vi "RegPatchGenerator.vi"(8 "error in":errorcluster, 9 "reg patch file":path=path "C:/Users/liyao/Desktop", 10 "extensions":string[](array[string])=[".lvproj", ".lvlib", ".lvlibp", ".vi", ".llb", ".ctl", ".lvclass", ".vit", ".xctl", ".lvsc", ".lvrbt", ".vim", ".lvtest", ".ctt"], 11 "exe path":path=path "C:/Users/liyao/Desktop/LabVIEW-Version-Selector/Build/LabVIEW Version Selector.exe") -> (0 "error out":errorcluster, 3 "install.reg":string="Windows Registry Editor Version 5.00\n\n[HKEY_CLASSES_ROOT\\Applications\\LabVIEW Version Selector.exe]\n\n[HKEY_CLASSES_ROOT\\Applications\\LabVIEW Version Selector.exe\\shell]\n\n[HKEY_CLASSES_ROOT\\Applications\\LabVIEW Version Selector.exe\\shell\\open]\n\n[HKEY_CLASSES_ROOT\\Applications\\LabVIEW Version Selector.exe\\shell\\open\\command]\n@=\"\\\"\"\"\" \"%1\"\"\\\" \\\"%1\\\"\"\n\n[HKEY_CURRENT_USER\\Software\\Classes\\Applications\\LabVIEW Version Selector.exe]\n\n[HKEY_CURRENT_USER\\Software\\Classes\\Applications\\LabVIEW Version Selector.exe\\shell]\n\n[HKEY_CURRENT_USER\\Software\\Classes\\Applications\\LabVIEW Version Selector.exe\\shell\\open]\n\n[HKEY_CURRENT_USER\\Software\\Classes\\Applications\\LabVIEW Version Selector.exe\\shell\\open\\command]\n@=\"\\\"\"\"\" \"%1\"\"\\\" \\\"%1\\\"\"\n\n[HKEY_CURRENT_USER\\Software\\Microsoft\\Windows\\CurrentVersion\\Explorer\\FileExts\\.lvproj\\OpenWithList]\n\"a\"=\"LabVIEW.exe\"\n\"b\"=\"LabVIEW Version Selector.exe\"\n\"MRUList\"=\"ba\"\n\n[HKEY_CURRENT_USER\\Software\\Microsoft\\Windows\\CurrentVersion\\Explorer\\FileExts\\.lvproj\\UserChoice]\n\"ProgId\"=\"Applications\\\\LabVIEW Version Selector.exe\"\n\n[HKEY_CLASSES_ROOT\\LabVIEWProject\r\n\\shell\\open\\command]\n@=\"\\\"\"\"\" \"%1\"\"\\\" \\\"%1\\\"\"\n\n[HKEY_LOCAL_MACHINE\\SOFTWARE\\Classes\\LabVIEWProject\r\n\\shell\\open\\command]\n@=hex(2):<HEXEXEPATH>\n\n[HKEY_CURRENT_USER\\Software\\Microsoft\\Windows\\CurrentVersion\\Explorer\\FileExts\\.lvlib\\OpenWithList]\n\"a\"=\"LabVIEW.exe\"\n\"b\"=\"LabVIEW Version Selector.exe\"\n\"MRUList\"=\"ba\"\n\n[HKEY_CURRENT_USER\\Software\\Microsoft\\Windows\\CurrentVersion\\Explorer\\FileExts\\.lvlib\\UserChoice]\n\"ProgId\"=\"Applications\\\\LabVIEW Version Selector.exe\"\n\n[HKEY_CLASSES_ROOT\\LabVIEWLabVIEW Library\r\n\\shell\\open\\command]\n@=\"\\\"\"\"\" \"%1\"\"\\\" \\\"%1\\\"\"\n\n[HKEY_LOCAL_MACHINE\\SOFTWARE\\Classes\\LabVIEWLabVIEW Library\r\n\\shell\\open\\command]\n@=hex(2):<HEXEXEPATH>\n\n[HKEY_CURRENT_USER\\Software\\Microsoft\\Windows\\CurrentVersion\\Explorer\\FileExts\\.lvlibp\\OpenWithList]\n\"a\"=\"LabVIEW.exe\"\n\"b\"=\"LabVIEW Version Selector.exe\"\n\"MRUList\"=\"ba\"\n\n[HKEY_CURRENT_USER\\Software\\Microsoft\\Windows\\CurrentVersion\\Explorer\\FileExts\\.lvlibp\\UserChoice]\n\"ProgId\"=\"Applications\\\\LabVIEW Version Selector.exe\"\n\n[HKEY_CLASSES_ROOT\\LabVIEWLabVIEW Packed Library\r\n\\shell\\open\\command]\n@=\"\\\"\"\"\" \"%1\"\"\\\" \\\"%1\\\"\"\n\n[HKEY_LOCAL_MACHINE\\SOFTWARE\\Classes\\LabVIEWLabVIEW Packed Library\r\n\\shell\\open\\command]\n@=hex(2):<HEXEXEPATH>\n\n[HKEY_CURRENT_USER\\Software\\Microsoft\\Windows\\CurrentVersion\\Explorer\\FileExts\\.vi\\OpenWithList]\n\"a\"=\"LabVIEW.exe\"\n\"b\"=\"LabVIEW Version Selector.exe\"\n\"MRUList\"=\"ba\"\n\n[HKEY_CURRENT_USER\\Software\\Microsoft\\Windows\\CurrentVersion\\Explorer\\FileExts\\.vi\\UserChoice]\n\"ProgId\"=\"Applications\\\\LabVIEW Version Selector.exe\"\n\n[HKEY_CLASSES_ROOT\\LabVIEWInstrument\r\n\\shell\\open\\command]\n@=\"\\\"\"\"\" \"%1\"\"\\\" \\\"%1\\\"\"\n\n[HKEY_LOCAL_MACHINE\\SOFTWARE\\Classes\\LabVIEWInstrument\r\n\\shell\\open\\command]\n@=hex(2):<HEXEXEPATH>\n\n[HKEY_CURRENT_USER\\Software\\Microsoft\\Windows\\CurrentVersion\\Explorer\\FileExts\\.llb\\OpenWithList]\n\"a\"=\"LabVIEW.exe\"\n\"b\"=\"LabVIEW Version Selector.exe\"\n\"MRUList\"=\"ba\"\n\n[HKEY_CURRENT_USER\\Software\\Microsoft\\Windows\\CurrentVersion\\Explorer\\FileExts\\.llb\\UserChoice]\n\"ProgId\"=\"Applications\\\\LabVIEW Version Selector.exe\"\n\n[HKEY_CLASSES_ROOT\\LabVIEWLibrary\r\n\\shell\\open\\command]\n@=\"\\\"\"\"\" \"%1\"\"\\\" \\\"%1\\\"\"\n\n[HKEY_LOCAL_MACHINE\\SOFTWARE\\Classes\\LabVIEWLibrary\r\n\\shell\\open\\command]\n@=hex(2):<HEXEXEPATH>\n\n[HKEY_CURRENT_USER\\Software\\Microsoft\\Windows\\CurrentVersion\\Explorer\\FileExts\\.ctl\\OpenWithList]\n\"a\"=\"LabVIEW.exe\"\n\"b\"=\"LabVIEW Version Selector.exe\"\n\"MRUList\"=\"ba\"\n\n[HKEY_CURRENT_USER\\Software\\Microsoft\\Windows\\CurrentVersion\\Explorer\\FileExts\\.ctl\\UserChoice]\n\"ProgId\"=\"Applications\\\\LabVIEW Version Selector.exe\"\n\n[HKEY_CLASSES_ROOT\\LabVIEWControl\r\n\\shell\\open\\command]\n@=\"\\\"\"\"\" \"%1\"\"\\\" \\\"%1\\\"\"\n\n[HKEY_LOCAL_MACHINE\\SOFTWARE\\Classes\\LabVIEWControl\r\n\\shell\\open\\command]\n@=hex(2):<HEXEXEPATH>\n\n[HKEY_CURRENT_USER\\Software\\Microsoft\\Windows\\CurrentVersion\\Explorer\\FileExts\\.lvclass\\OpenWithList]\n\"a\"=\"LabVIEW.exe\"\n\"b\"=\"LabVIEW Version Selector.exe\"\n\"MRUList\"=\"ba\"\n\n[HKEY_CURRENT_USER\\Software\\Microsoft\\Windows\\CurrentVersion\\Explorer\\FileExts\\.lvclass\\UserChoice]\n\"ProgId\"=\"Applications\\\\LabVIEW Version Selector.exe\"\n\n[HKEY_CLASSES_ROOT\\LabVIEWLabVIEW Class\r\n\\shell\\open\\command]\n@=\"\\\"\"\"\" \"%1\"\"\\\" \\\"%1\\\"\"\n\n[HKEY_LOCAL_MACHINE\\SOFTWARE\\Classes\\LabVIEWLabVIEW Class\r\n\\shell\\open\\command]\n@=hex(2):<HEXEXEPATH>\n\n[HKEY_CURRENT_USER\\Software\\Microsoft\\Windows\\CurrentVersion\\Explorer\\FileExts\\.vit\\OpenWithList]\n\"a\"=\"LabVIEW.exe\"\n\"b\"=\"LabVIEW Version Selector.exe\"\n\"MRUList\"=\"ba\"\n\n[HKEY_CURRENT_USER\\Software\\Microsoft\\Windows\\CurrentVersion\\Explorer\\FileExts\\.vit\\UserChoice]\n\"ProgId\"=\"Applications\\\\LabVIEW Version Selector.exe\"\n\n[HKEY_CLASSES_ROOT\\LabVIEWInstrumentTemplate\r\n\\shell\\open\\command]\n@=\"\\\"\"\"\" \"%1\"\"\\\" \\\"%1\\\"\"\n\n[HKEY_LOCAL_MACHINE\\SOFTWARE\\Classes\\LabVIEWInstrumentTemplate\r\n\\shell\\open\\command]\n@=hex(2):<HEXEXEPATH>\n\n[HKEY_CURRENT_USER\\Software\\Microsoft\\Windows\\CurrentVersion\\Explorer\\FileExts\\.xctl\\OpenWithList]\n\"a\"=\"LabVIEW.exe\"\n\"b\"=\"LabVIEW Version Selector.exe\"\n\"MRUList\"=\"ba\"\n\n[HKEY_CURRENT_USER\\Software\\Microsoft\\Windows\\CurrentVersion\\Explorer\\FileExts\\.xctl\\UserChoice]\n\"ProgId\"=\"Applications\\\\LabVIEW Version Selector.exe\"\n\n[HKEY_CLASSES_ROOT\\LabVIEWXControl\r\n\\shell\\open\\command]\n@=\"\\\"\"\"\" \"%1\"\"\\\" \\\"%1\\\"\"\n\n[HKEY_LOCAL_MACHINE\\SOFTWARE\\Classes\\LabVIEWXControl\r\n\\shell\\open\\command]\n@=hex(2):<HEXEXEPATH>\n\n[HKEY_CURRENT_USER\\Software\\Microsoft\\Windows\\CurrentVersion\\Explorer\\FileExts\\.lvtest\\OpenWithList]\n\"a\"=\"LabVIEW.exe\"\n\"b\"=\"LabVIEW Version Selector.exe\"\n\"MRUList\"=\"ba\"\n\n[HKEY_CURRENT_USER\\Software\\Microsoft\\Windows\\CurrentVersion\\Explorer\\FileExts\\.lvtest\\UserChoice]\n\"ProgId\"=\"Applications\\\\LabVIEW Version Selector.exe\"\n\n[HKEY_CLASSES_ROOT\\\\shell\\open\\command]\n@=\"\\\"\"\"\" \"%1\"\"\\\" \\\"%1\\\"\"\n\n[HKEY_LOCAL_MACHINE\\SOFTWARE\\Classes\\\\shell\\open\\command]\n@=hex(2):<HEXEXEPATH>\n\n[HKEY_CURRENT_USER\\Software\\Microsoft\\Windows\\CurrentVersion\\Explorer\\FileExts\\.lvvect\\OpenWithList]\n\"a\"=\"LabVIEW.exe\"\n\"b\"=\"LabVIEW Version Selector.exe\"\n\"MRUList\"=\"ba\"\n\n[HKEY_CURRENT_USER\\Software\\Microsoft\\Windows\\CurrentVersion\\Explorer\\FileExts\\.lvvect\\UserChoice]\n\"ProgId\"=\"Applications\\\\LabVIEW Version Selector.exe\"\n\n[HKEY_CLASSES_ROOT\\\\shell\\open\\command]\n@=\"\\\"\"\"\" \"%1\"\"\\\" \\\"%1\\\"\"\n\n[HKEY_LOCAL_MACHINE\\SOFTWARE\\Classes\\\\shell\\open\\command]\n@=hex(2):<HEXEXEPATH>\n\n[HKEY_CURRENT_USER\\Software\\Microsoft\\Windows\\CurrentVersion\\Explorer\\FileExts\\.lvsc\\OpenWithList]\n\"a\"=\"LabVIEW.exe\"\n\"b\"=\"LabVIEW Version Selector.exe\"\n\"MRUList\"=\"ba\"\n\n[HKEY_CURRENT_USER\\Software\\Microsoft\\Windows\\CurrentVersion\\Explorer\\FileExts\\.lvsc\\UserChoice]\n\"ProgId\"=\"Applications\\\\LabVIEW Version Selector.exe\"\n\n[HKEY_CLASSES_ROOT\\LabVIEW Statechart\r\n\\shell\\open\\command]\n@=\"\\\"\"\"\" \"%1\"\"\\\" \\\"%1\\\"\"\n\n[HKEY_LOCAL_MACHINE\\SOFTWARE\\Classes\\LabVIEW Statechart\r\n\\shell\\open\\command]\n@=hex(2):<HEXEXEPATH>\n\n[HKEY_CURRENT_USER\\Software\\Microsoft\\Windows\\CurrentVersion\\Explorer\\FileExts\\.LVCLASS\\OpenWithList]\n\"a\"=\"LabVIEW.exe\"\n\"b\"=\"LabVIEW Version Selector.exe\"\n\"MRUList\"=\"ba\"\n\n[HKEY_CURRENT_USER\\Software\\Microsoft\\Windows\\CurrentVersion\\Explorer\\FileExts\\.LVCLASS\\UserChoice]\n\"ProgId\"=\"Applications\\\\LabVIEW Version Selector.exe\"\n\n[HKEY_CLASSES_ROOT\\LabVIEWLabVIEW Class\r\n\\shell\\open\\command]\n@=\"\\\"\"\"\" \"%1\"\"\\\" \\\"%1\\\"\"\n\n[HKEY_LOCAL_MACHINE\\SOFTWARE\\Classes\\LabVIEWLabVIEW Class\r\n\\shell\\open\\command]\n@=hex(2):<HEXEXEPATH>\n\n[HKEY_CURRENT_USER\\Software\\Microsoft\\Windows\\CurrentVersion\\Explorer\\FileExts\\.lvr\\OpenWithList]\n\"a\"=\"LabVIEW.exe\"\n\"b\"=\"LabVIEW Version Selector.exe\"\n\"MRUList\"=\"ba\"\n\n[HKEY_CURRENT_USER\\Software\\Microsoft\\Windows\\CurrentVersion\\Explorer\\FileExts\\.lvr\\UserChoice]\n\"ProgId\"=\"Applications\\\\LabVIEW Version Selector.exe\"\n\n[HKEY_CLASSES_ROOT\\\\shell\\open\\command]\n@=\"\\\"\"\"\" \"%1\"\"\\\" \\\"%1\\\"\"\n\n[HKEY_LOCAL_MACHINE\\SOFTWARE\\Classes\\\\shell\\open\\command]\n@=hex(2):<HEXEXEPATH>\n\n[HKEY_CURRENT_USER\\Software\\Microsoft\\Windows\\CurrentVersion\\Explorer\\FileExts\\.lvrbt\\OpenWithList]\n\"a\"=\"LabVIEW.exe\"\n\"b\"=\"LabVIEW Version Selector.exe\"\n\"MRUList\"=\"ba\"\n\n[HKEY_CURRENT_USER\\Software\\Microsoft\\Windows\\CurrentVersion\\Explorer\\FileExts\\.lvrbt\\UserChoice]\n\"ProgId\"=\"Applications\\\\LabVIEW Version Selector.exe\"\n\n[HKEY_CLASSES_ROOT\\LabVIEWNXTRobotProject\r\n\\shell\\open\\command]\n@=\"\\\"\"\"\" \"%1\"\"\\\" \\\"%1\\\"\"\n\n[HKEY_LOCAL_MACHINE\\SOFTWARE\\Classes\\LabVIEWNXTRobotProject\r\n\\shell\\open\\command]\n@=hex(2):<HEXEXEPATH>")   [LabVIEW 2014]
uses:
  <userlib>/_OpenG.lib/array/array.llb/Remove Duplicates from 1D Array (String)__ogtk.vi
panel:
  out "unstall.reg":string="Windows Registry Editor Version 5.00\n\n[HKEY_CLASSES_ROOT\\Applications\\LabVIEW Version Selector.exe]\n\n[HKEY_CLASSES_ROOT\\Applications\\LabVIEW Version Selector.exe\\shell]\n\n[HKEY_CLASSES_ROOT\\Applications\\LabVIEW Version Selector.exe\\shell\\open]\n\n[HKEY_CLASSES_ROOT\\Applications\\LabVIEW Version Selector.exe\\shell\\open\\command]\n@=\"\\\"\"\"\" \"%1\"\"\\\" \\\"%1\\\"\"\n\n[HKEY_CURRENT_USER\\Software\\Classes\\Applications\\LabVIEW Version Selector.exe]\n\n[HKEY_CURRENT_USER\\Software\\Classes\\Applications\\LabVIEW Version Selector.exe\\shell]\n\n[HKEY_CURRENT_USER\\Software\\Classes\\Applications\\LabVIEW Version Selector.exe\\shell\\open]\n\n[HKEY_CURRENT_USER\\Software\\Classes\\Applications\\LabVIEW Version Selector.exe\\shell\\open\\command]\n@=\"\\\"\"\"\" \"%1\"\"\\\" \\\"%1\\\"\"\n\n[HKEY_CURRENT_USER\\Software\\Microsoft\\Windows\\CurrentVersion\\Explorer\\FileExts\\.lvproj\\OpenWithList]\n\"a\"=\"LabVIEW.exe\"\n\"b\"=\"LabVIEW Version Selector.exe\"\n\"MRUList\"=\"ba\"\n\n[HKEY_CURRENT_USER\\Software\\Microsoft\\Windows\\CurrentVersion\\Explorer\\FileExts\\.lvproj\\UserChoice]\n\"ProgId\"=\"Applications\\\\LabVIEW Version Selector.exe\"\n\n[HKEY_CLASSES_ROOT\\LabVIEWProject\r\n\\shell\\open\\command]\n@=\"\\\"\"\"\" \"%1\"\"\\\" \\\"%1\\\"\"\n\n[HKEY_LOCAL_MACHINE\\SOFTWARE\\Classes\\LabVIEWProject\r\n\\shell\\open\\command]\n@=hex(2):<HEXEXEPATH>\n\n[HKEY_CURRENT_USER\\Software\\Microsoft\\Windows\\CurrentVersion\\Explorer\\FileExts\\.lvlib\\OpenWithList]\n\"a\"=\"LabVIEW.exe\"\n\"b\"=\"LabVIEW Version Selector.exe\"\n\"MRUList\"=\"ba\"\n\n[HKEY_CURRENT_USER\\Software\\Microsoft\\Windows\\CurrentVersion\\Explorer\\FileExts\\.lvlib\\UserChoice]\n\"ProgId\"=\"Applications\\\\LabVIEW Version Selector.exe\"\n\n[HKEY_CLASSES_ROOT\\LabVIEWLabVIEW Library\r\n\\shell\\open\\command]\n@=\"\\\"\"\"\" \"%1\"\"\\\" \\\"%1\\\"\"\n\n[HKEY_LOCAL_MACHINE\\SOFTWARE\\Classes\\LabVIEWLabVIEW Library\r\n\\shell\\open\\command]\n@=hex(2):<HEXEXEPATH>\n\n[HKEY_CURRENT_USER\\Software\\Microsoft\\Windows\\CurrentVersion\\Explorer\\FileExts\\.lvlibp\\OpenWithList]\n\"a\"=\"LabVIEW.exe\"\n\"b\"=\"LabVIEW Version Selector.exe\"\n\"MRUList\"=\"ba\"\n\n[HKEY_CURRENT_USER\\Software\\Microsoft\\Windows\\CurrentVersion\\Explorer\\FileExts\\.lvlibp\\UserChoice]\n\"ProgId\"=\"Applications\\\\LabVIEW Version Selector.exe\"\n\n[HKEY_CLASSES_ROOT\\LabVIEWLabVIEW Packed Library\r\n\\shell\\open\\command]\n@=\"\\\"\"\"\" \"%1\"\"\\\" \\\"%1\\\"\"\n\n[HKEY_LOCAL_MACHINE\\SOFTWARE\\Classes\\LabVIEWLabVIEW Packed Library\r\n\\shell\\open\\command]\n@=hex(2):<HEXEXEPATH>\n\n[HKEY_CURRENT_USER\\Software\\Microsoft\\Windows\\CurrentVersion\\Explorer\\FileExts\\.vi\\OpenWithList]\n\"a\"=\"LabVIEW.exe\"\n\"b\"=\"LabVIEW Version Selector.exe\"\n\"MRUList\"=\"ba\"\n\n[HKEY_CURRENT_USER\\Software\\Microsoft\\Windows\\CurrentVersion\\Explorer\\FileExts\\.vi\\UserChoice]\n\"ProgId\"=\"Applications\\\\LabVIEW Version Selector.exe\"\n\n[HKEY_CLASSES_ROOT\\LabVIEWInstrument\r\n\\shell\\open\\command]\n@=\"\\\"\"\"\" \"%1\"\"\\\" \\\"%1\\\"\"\n\n[HKEY_LOCAL_MACHINE\\SOFTWARE\\Classes\\LabVIEWInstrument\r\n\\shell\\open\\command]\n@=hex(2):<HEXEXEPATH>\n\n[HKEY_CURRENT_USER\\Software\\Microsoft\\Windows\\CurrentVersion\\Explorer\\FileExts\\.llb\\OpenWithList]\n\"a\"=\"LabVIEW.exe\"\n\"b\"=\"LabVIEW Version Selector.exe\"\n\"MRUList\"=\"ba\"\n\n[HKEY_CURRENT_USER\\Software\\Microsoft\\Windows\\CurrentVersion\\Explorer\\FileExts\\.llb\\UserChoice]\n\"ProgId\"=\"Applications\\\\LabVIEW Version Selector.exe\"\n\n[HKEY_CLASSES_ROOT\\LabVIEWLibrary\r\n\\shell\\open\\command]\n@=\"\\\"\"\"\" \"%1\"\"\\\" \\\"%1\\\"\"\n\n[HKEY_LOCAL_MACHINE\\SOFTWARE\\Classes\\LabVIEWLibrary\r\n\\shell\\open\\command]\n@=hex(2):<HEXEXEPATH>\n\n[HKEY_CURRENT_USER\\Software\\Microsoft\\Windows\\CurrentVersion\\Explorer\\FileExts\\.ctl\\OpenWithList]\n\"a\"=\"LabVIEW.exe\"\n\"b\"=\"LabVIEW Version Selector.exe\"\n\"MRUList\"=\"ba\"\n\n[HKEY_CURRENT_USER\\Software\\Microsoft\\Windows\\CurrentVersion\\Explorer\\FileExts\\.ctl\\UserChoice]\n\"ProgId\"=\"Applications\\\\LabVIEW Version Selector.exe\"\n\n[HKEY_CLASSES_ROOT\\LabVIEWControl\r\n\\shell\\open\\command]\n@=\"\\\"\"\"\" \"%1\"\"\\\" \\\"%1\\\"\"\n\n[HKEY_LOCAL_MACHINE\\SOFTWARE\\Classes\\LabVIEWControl\r\n\\shell\\open\\command]\n@=hex(2):<HEXEXEPATH>\n\n[HKEY_CURRENT_USER\\Software\\Microsoft\\Windows\\CurrentVersion\\Explorer\\FileExts\\.lvclass\\OpenWithList]\n\"a\"=\"LabVIEW.exe\"\n\"b\"=\"LabVIEW Version Selector.exe\"\n\"MRUList\"=\"ba\"\n\n[HKEY_CURRENT_USER\\Software\\Microsoft\\Windows\\CurrentVersion\\Explorer\\FileExts\\.lvclass\\UserChoice]\n\"ProgId\"=\"Applications\\\\LabVIEW Version Selector.exe\"\n\n[HKEY_CLASSES_ROOT\\LabVIEWLabVIEW Class\r\n\\shell\\open\\command]\n@=\"\\\"\"\"\" \"%1\"\"\\\" \\\"%1\\\"\"\n\n[HKEY_LOCAL_MACHINE\\SOFTWARE\\Classes\\LabVIEWLabVIEW Class\r\n\\shell\\open\\command]\n@=hex(2):<HEXEXEPATH>\n\n[HKEY_CURRENT_USER\\Software\\Microsoft\\Windows\\CurrentVersion\\Explorer\\FileExts\\.vit\\OpenWithList]\n\"a\"=\"LabVIEW.exe\"\n\"b\"=\"LabVIEW Version Selector.exe\"\n\"MRUList\"=\"ba\"\n\n[HKEY_CURRENT_USER\\Software\\Microsoft\\Windows\\CurrentVersion\\Explorer\\FileExts\\.vit\\UserChoice]\n\"ProgId\"=\"Applications\\\\LabVIEW Version Selector.exe\"\n\n[HKEY_CLASSES_ROOT\\LabVIEWInstrumentTemplate\r\n\\shell\\open\\command]\n@=\"\\\"\"\"\" \"%1\"\"\\\" \\\"%1\\\"\"\n\n[HKEY_LOCAL_MACHINE\\SOFTWARE\\Classes\\LabVIEWInstrumentTemplate\r\n\\shell\\open\\command]\n@=hex(2):<HEXEXEPATH>\n\n[HKEY_CURRENT_USER\\Software\\Microsoft\\Windows\\CurrentVersion\\Explorer\\FileExts\\.xctl\\OpenWithList]\n\"a\"=\"LabVIEW.exe\"\n\"b\"=\"LabVIEW Version Selector.exe\"\n\"MRUList\"=\"ba\"\n\n[HKEY_CURRENT_USER\\Software\\Microsoft\\Windows\\CurrentVersion\\Explorer\\FileExts\\.xctl\\UserChoice]\n\"ProgId\"=\"Applications\\\\LabVIEW Version Selector.exe\"\n\n[HKEY_CLASSES_ROOT\\LabVIEWXControl\r\n\\shell\\open\\command]\n@=\"\\\"\"\"\" \"%1\"\"\\\" \\\"%1\\\"\"\n\n[HKEY_LOCAL_MACHINE\\SOFTWARE\\Classes\\LabVIEWXControl\r\n\\shell\\open\\command]\n@=hex(2):<HEXEXEPATH>\n\n[HKEY_CURRENT_USER\\Software\\Microsoft\\Windows\\CurrentVersion\\Explorer\\FileExts\\.lvtest\\OpenWithList]\n\"a\"=\"LabVIEW.exe\"\n\"b\"=\"LabVIEW Version Selector.exe\"\n\"MRUList\"=\"ba\"\n\n[HKEY_CURRENT_USER\\Software\\Microsoft\\Windows\\CurrentVersion\\Explorer\\FileExts\\.lvtest\\UserChoice]\n\"ProgId\"=\"Applications\\\\LabVIEW Version Selector.exe\"\n\n[HKEY_CLASSES_ROOT\\\\shell\\open\\command]\n@=\"\\\"\"\"\" \"%1\"\"\\\" \\\"%1\\\"\"\n\n[HKEY_LOCAL_MACHINE\\SOFTWARE\\Classes\\\\shell\\open\\command]\n@=hex(2):<HEXEXEPATH>\n\n[HKEY_CURRENT_USER\\Software\\Microsoft\\Windows\\CurrentVersion\\Explorer\\FileExts\\.lvvect\\OpenWithList]\n\"a\"=\"LabVIEW.exe\"\n\"b\"=\"LabVIEW Version Selector.exe\"\n\"MRUList\"=\"ba\"\n\n[HKEY_CURRENT_USER\\Software\\Microsoft\\Windows\\CurrentVersion\\Explorer\\FileExts\\.lvvect\\UserChoice]\n\"ProgId\"=\"Applications\\\\LabVIEW Version Selector.exe\"\n\n[HKEY_CLASSES_ROOT\\\\shell\\open\\command]\n@=\"\\\"\"\"\" \"%1\"\"\\\" \\\"%1\\\"\"\n\n[HKEY_LOCAL_MACHINE\\SOFTWARE\\Classes\\\\shell\\open\\command]\n@=hex(2):<HEXEXEPATH>\n\n[HKEY_CURRENT_USER\\Software\\Microsoft\\Windows\\CurrentVersion\\Explorer\\FileExts\\.lvsc\\OpenWithList]\n\"a\"=\"LabVIEW.exe\"\n\"b\"=\"LabVIEW Version Selector.exe\"\n\"MRUList\"=\"ba\"\n\n[HKEY_CURRENT_USER\\Software\\Microsoft\\Windows\\CurrentVersion\\Explorer\\FileExts\\.lvsc\\UserChoice]\n\"ProgId\"=\"Applications\\\\LabVIEW Version Selector.exe\"\n\n[HKEY_CLASSES_ROOT\\LabVIEW Statechart\r\n\\shell\\open\\command]\n@=\"\\\"\"\"\" \"%1\"\"\\\" \\\"%1\\\"\"\n\n[HKEY_LOCAL_MACHINE\\SOFTWARE\\Classes\\LabVIEW Statechart\r\n\\shell\\open\\command]\n@=hex(2):<HEXEXEPATH>\n\n[HKEY_CURRENT_USER\\Software\\Microsoft\\Windows\\CurrentVersion\\Explorer\\FileExts\\.LVCLASS\\OpenWithList]\n\"a\"=\"LabVIEW.exe\"\n\"b\"=\"LabVIEW Version Selector.exe\"\n\"MRUList\"=\"ba\"\n\n[HKEY_CURRENT_USER\\Software\\Microsoft\\Windows\\CurrentVersion\\Explorer\\FileExts\\.LVCLASS\\UserChoice]\n\"ProgId\"=\"Applications\\\\LabVIEW Version Selector.exe\"\n\n[HKEY_CLASSES_ROOT\\LabVIEWLabVIEW Class\r\n\\shell\\open\\command]\n@=\"\\\"\"\"\" \"%1\"\"\\\" \\\"%1\\\"\"\n\n[HKEY_LOCAL_MACHINE\\SOFTWARE\\Classes\\LabVIEWLabVIEW Class\r\n\\shell\\open\\command]\n@=hex(2):<HEXEXEPATH>\n\n[HKEY_CURRENT_USER\\Software\\Microsoft\\Windows\\CurrentVersion\\Explorer\\FileExts\\.lvr\\OpenWithList]\n\"a\"=\"LabVIEW.exe\"\n\"b\"=\"LabVIEW Version Selector.exe\"\n\"MRUList\"=\"ba\"\n\n[HKEY_CURRENT_USER\\Software\\Microsoft\\Windows\\CurrentVersion\\Explorer\\FileExts\\.lvr\\UserChoice]\n\"ProgId\"=\"Applications\\\\LabVIEW Version Selector.exe\"\n\n[HKEY_CLASSES_ROOT\\\\shell\\open\\command]\n@=\"\\\"\"\"\" \"%1\"\"\\\" \\\"%1\\\"\"\n\n[HKEY_LOCAL_MACHINE\\SOFTWARE\\Classes\\\\shell\\open\\command]\n@=hex(2):<HEXEXEPATH>\n\n[HKEY_CURRENT_USER\\Software\\Microsoft\\Windows\\CurrentVersion\\Explorer\\FileExts\\.lvrbt\\OpenWithList]\n\"a\"=\"LabVIEW.exe\"\n\"b\"=\"LabVIEW Version Selector.exe\"\n\"MRUList\"=\"ba\"\n\n[HKEY_CURRENT_USER\\Software\\Microsoft\\Windows\\CurrentVersion\\Explorer\\FileExts\\.lvrbt\\UserChoice]\n\"ProgId\"=\"Applications\\\\LabVIEW Version Selector.exe\"\n\n[HKEY_CLASSES_ROOT\\LabVIEWNXTRobotProject\r\n\\shell\\open\\command]\n@=\"\\\"\"\"\" \"%1\"\"\\\" \\\"%1\\\"\"\n\n[HKEY_LOCAL_MACHINE\\SOFTWARE\\Classes\\LabVIEWNXTRobotProject\r\n\\shell\\open\\command]\n@=hex(2):<HEXEXEPATH>"
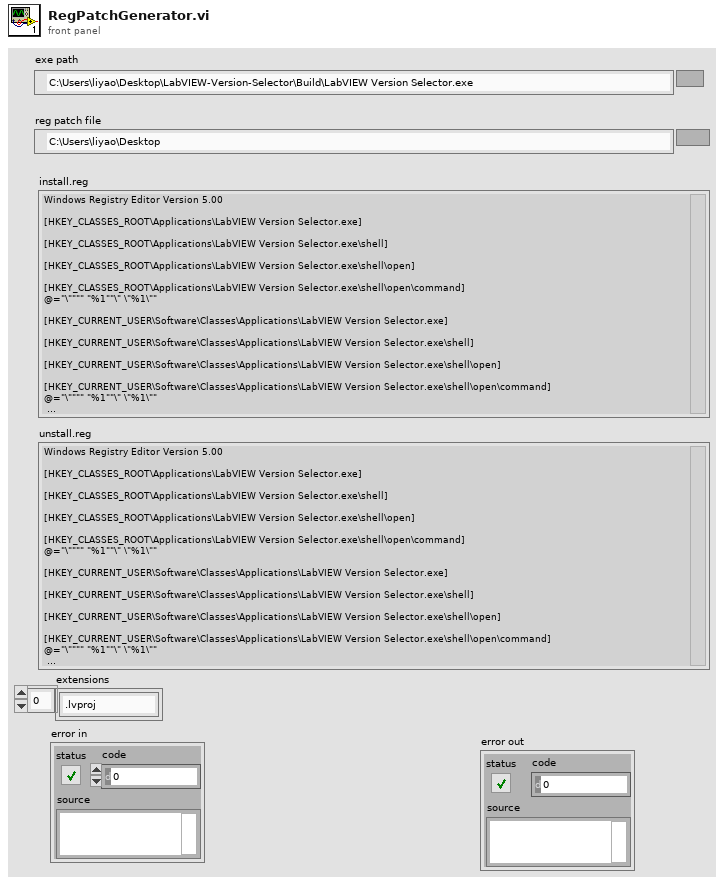
[diagram p1: front panel]
types:
  T1 = cluster{"dotEXT":string, "EXTTYPE":string[], "accoc":string}
  T2 = enum16{"open", "replace", "create", "open or create", "replace or create", "replace or create with confirmation"}
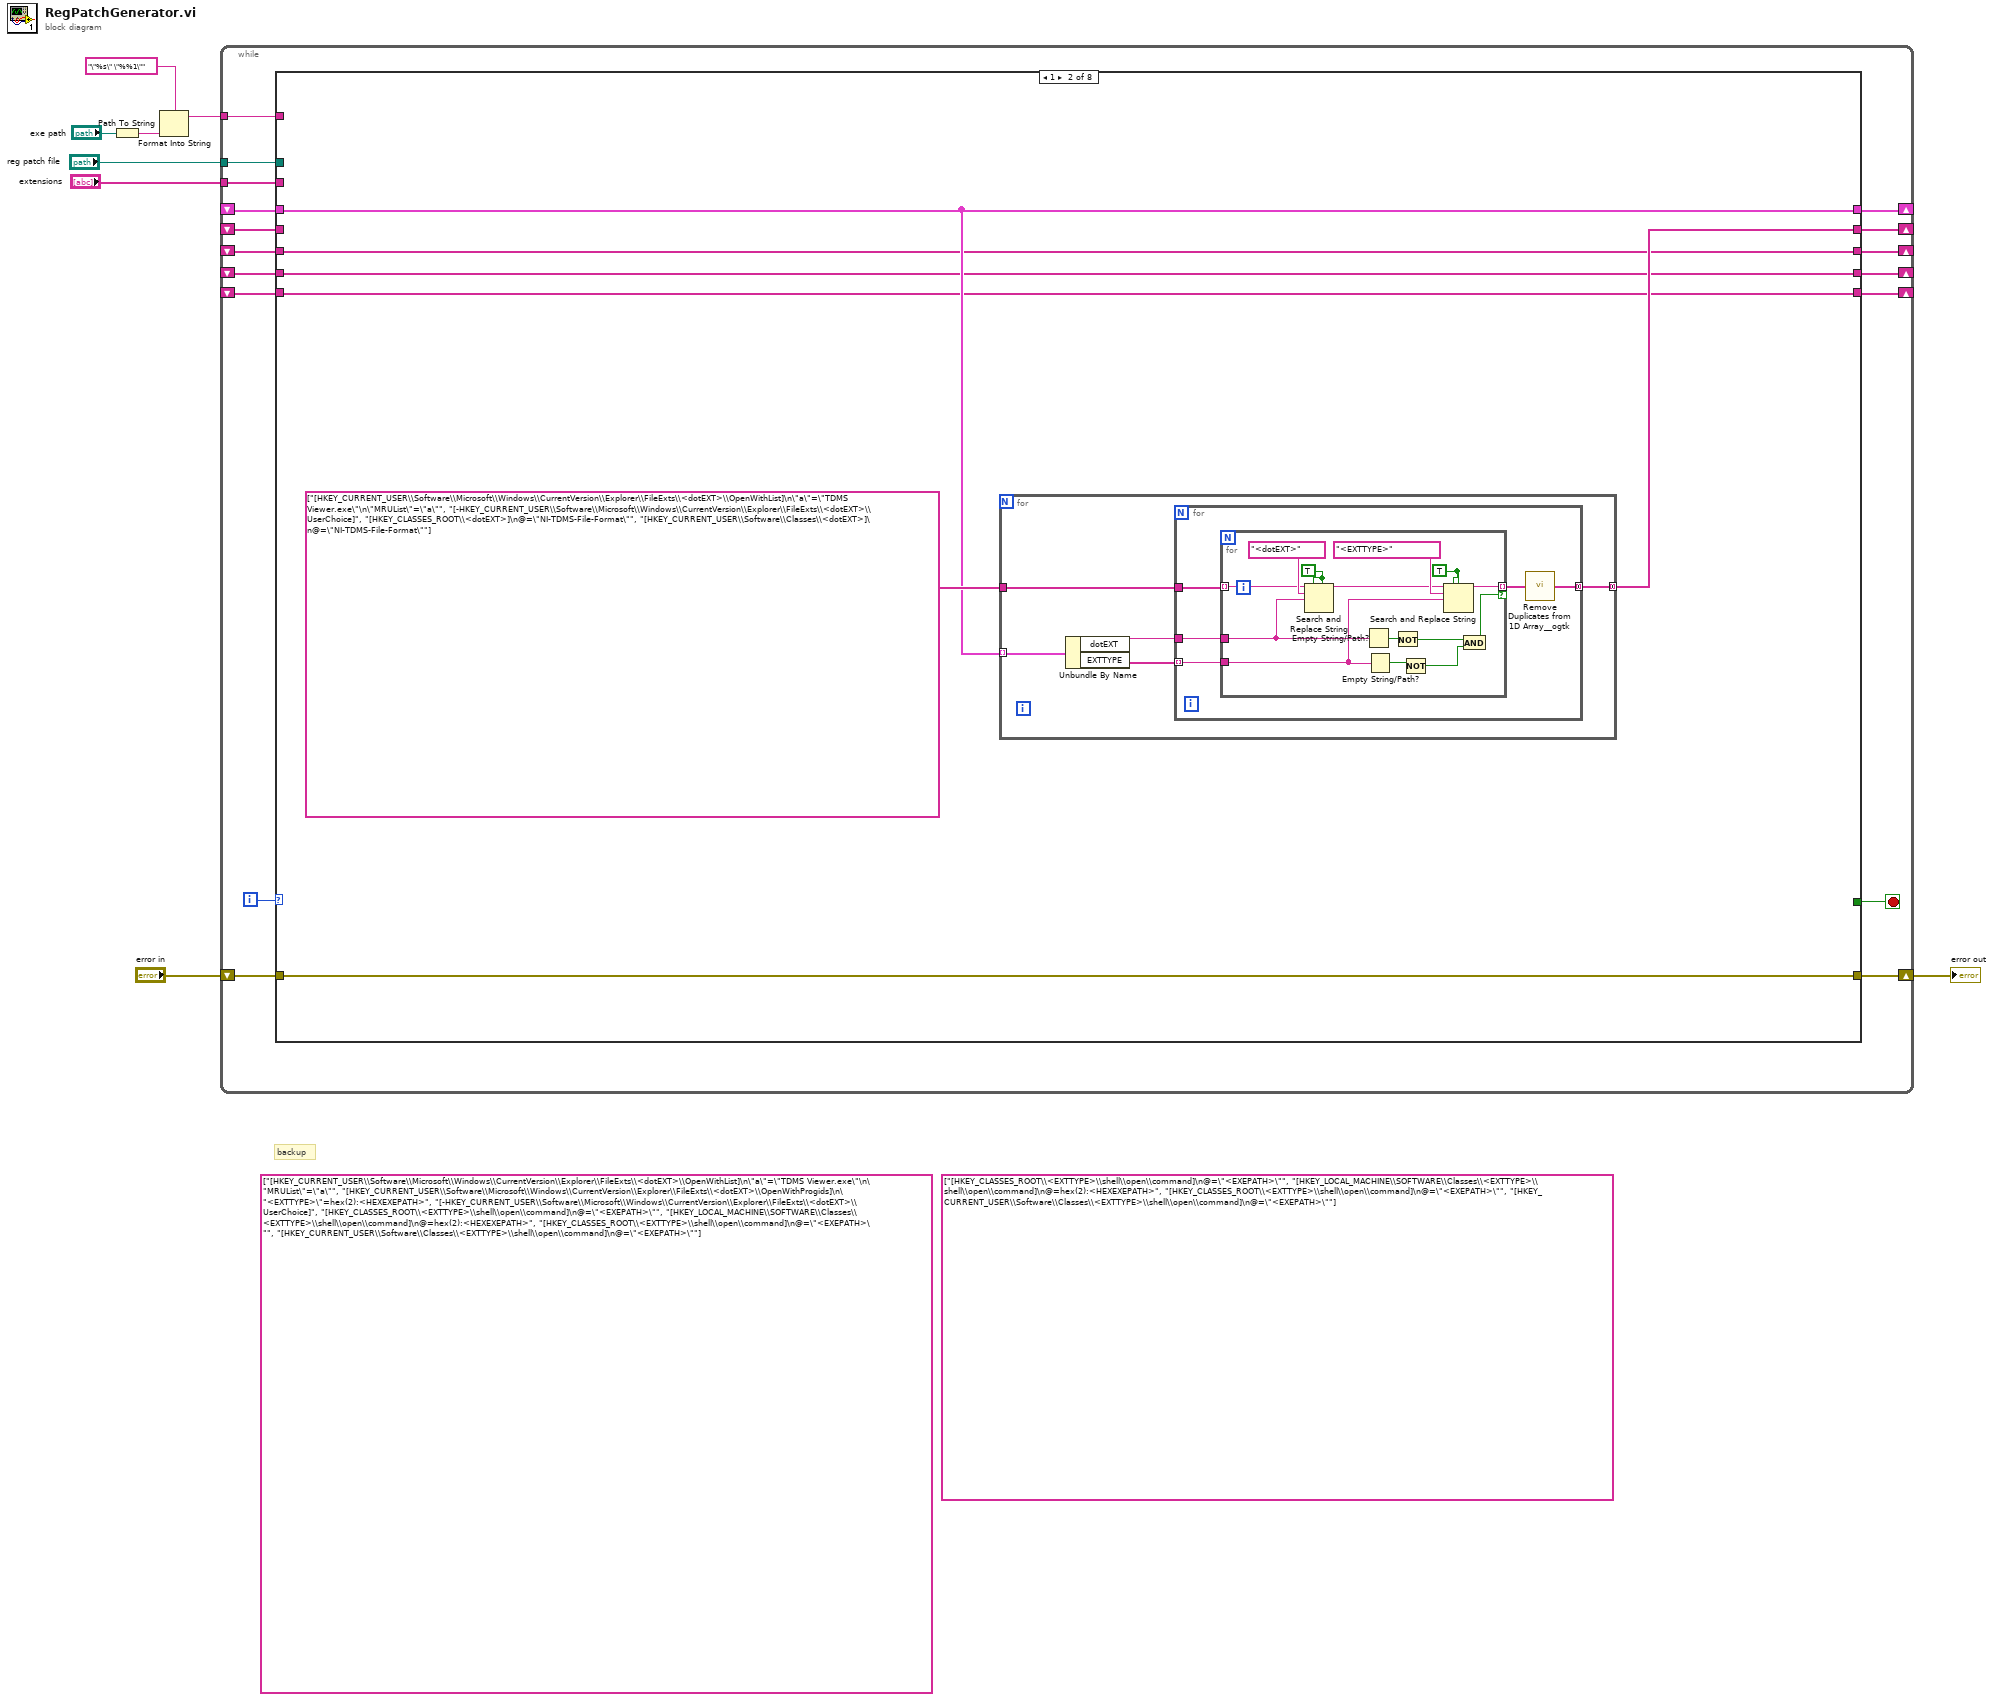
[diagram p0: block diagram]
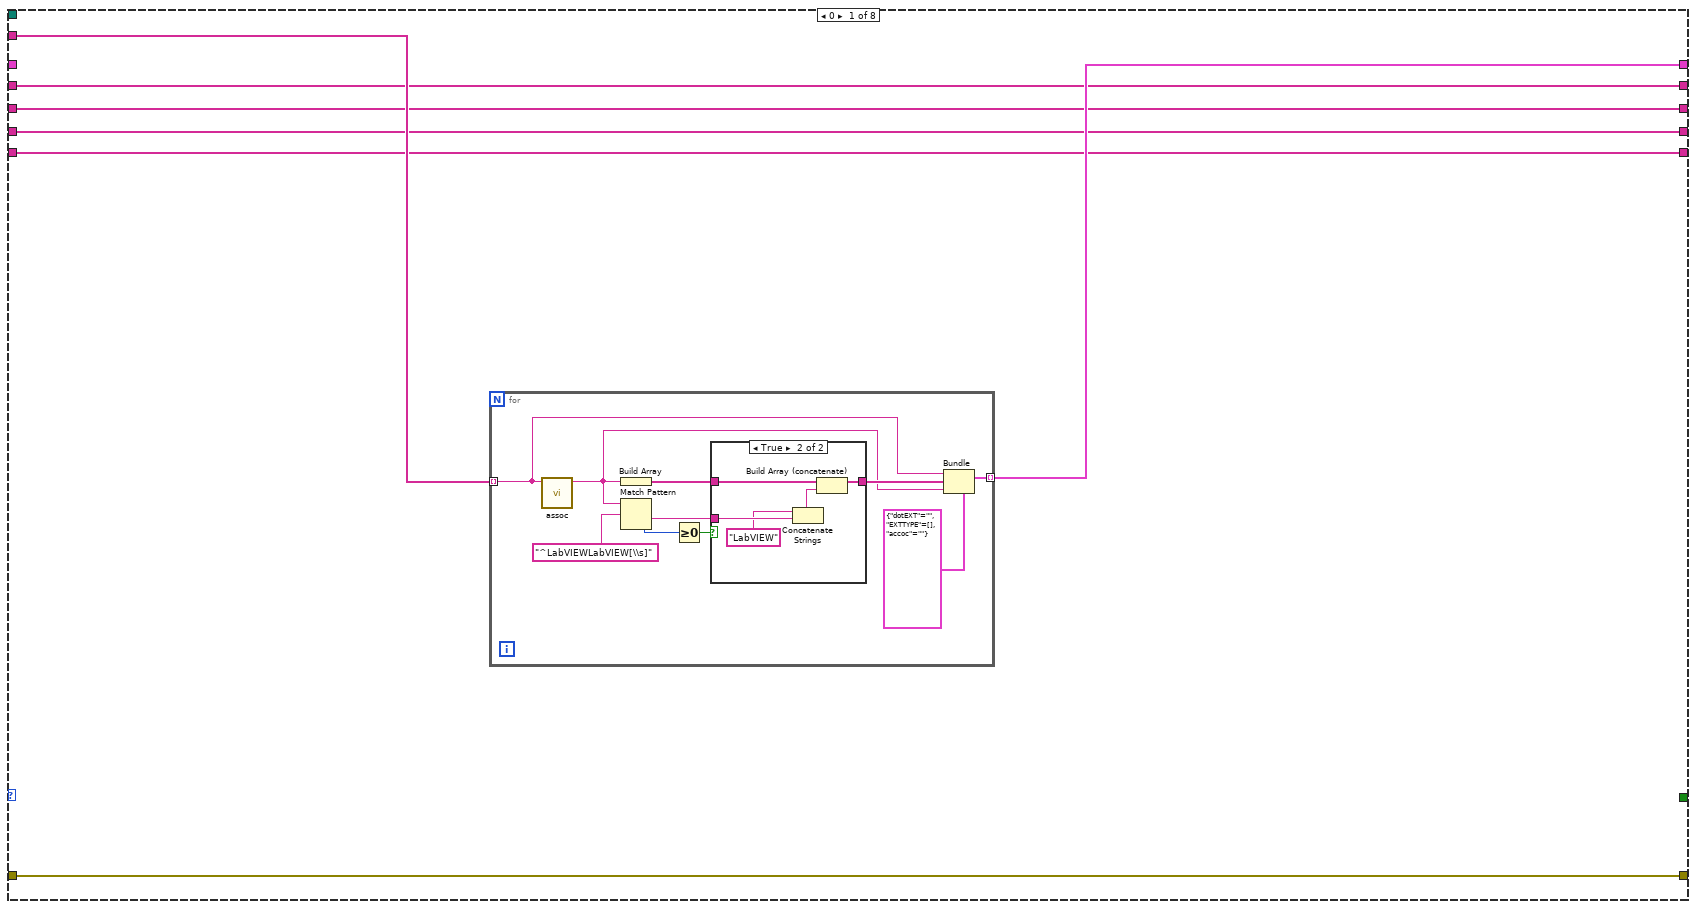
[diagram p2: hidden frame]
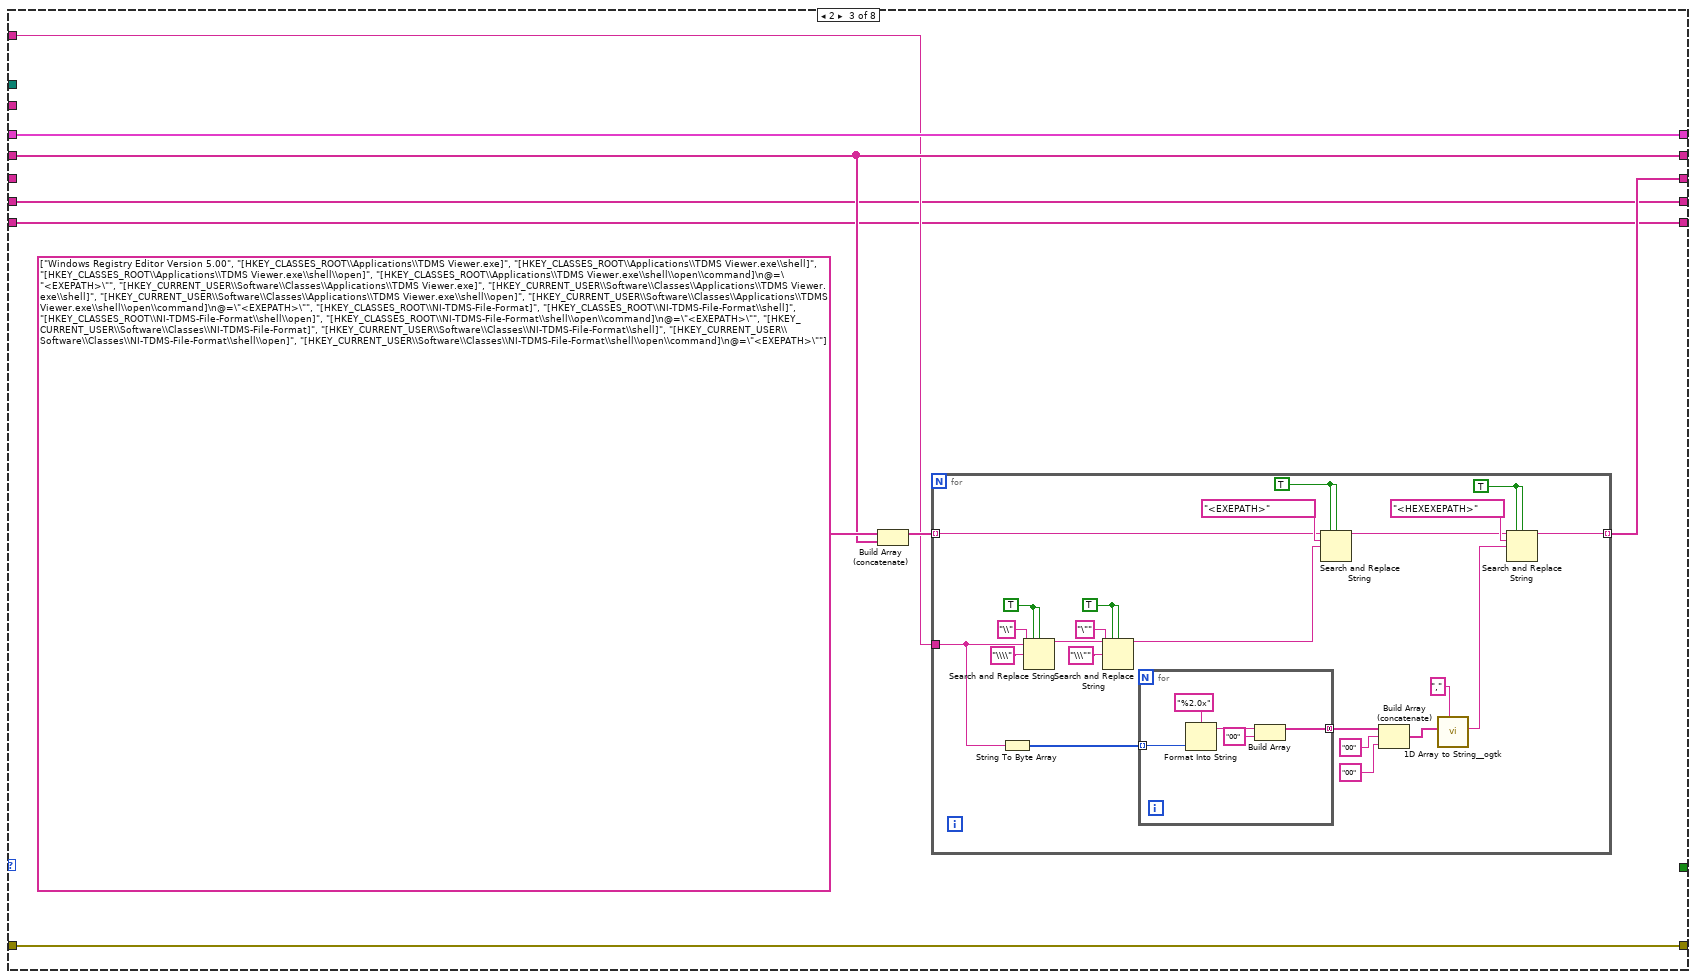
[diagram p4: hidden frame]
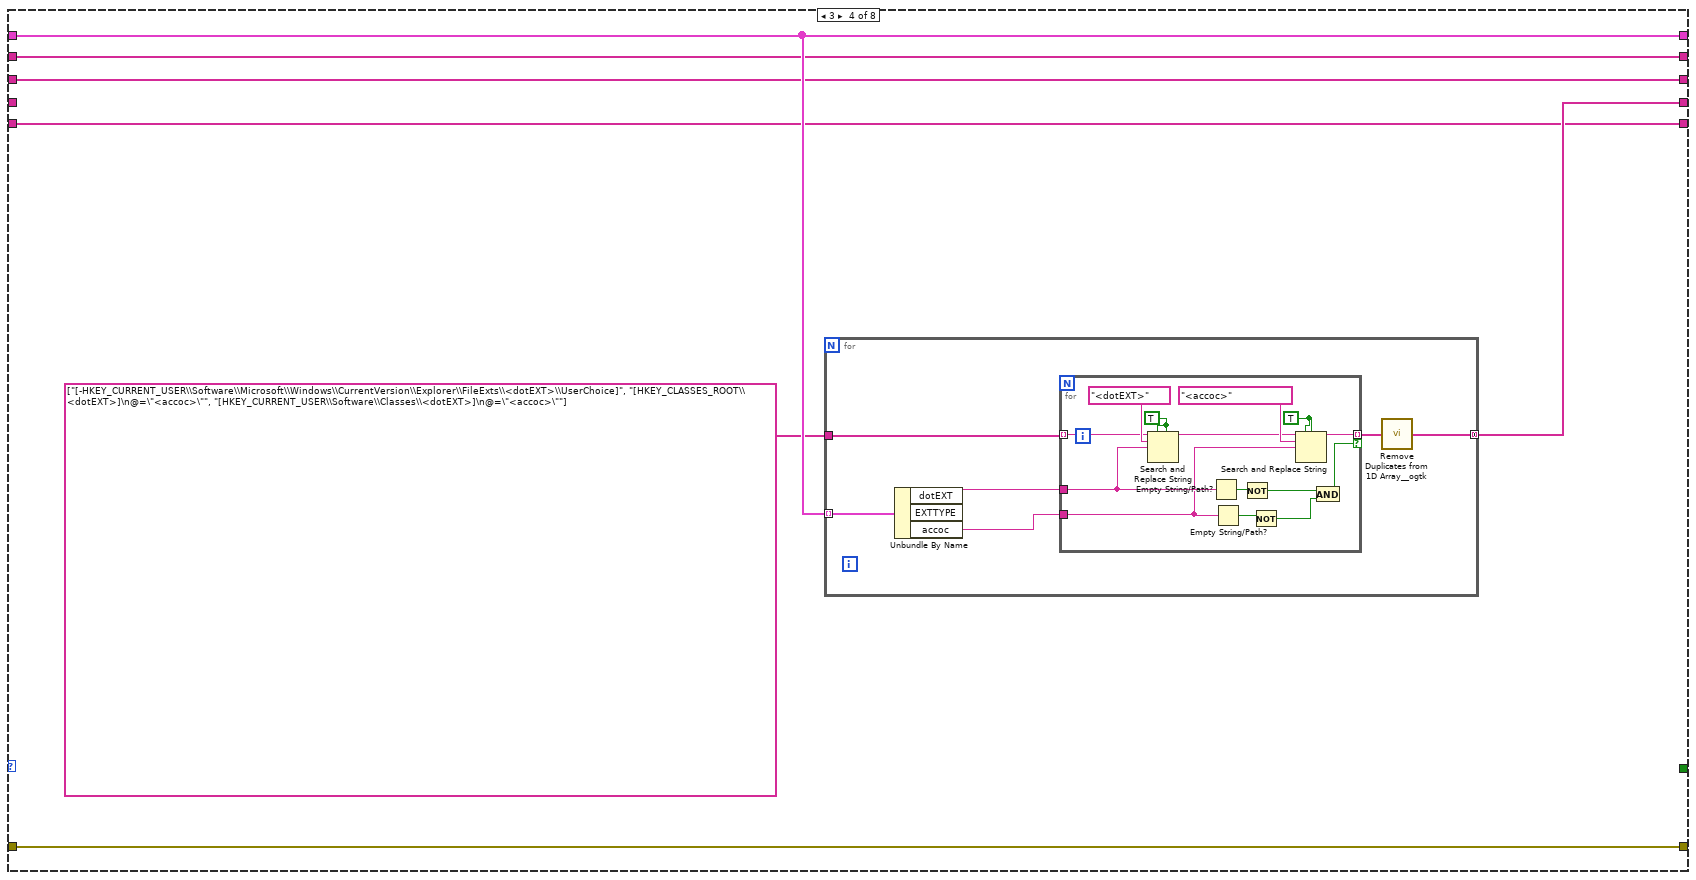
[diagram p5: hidden frame]
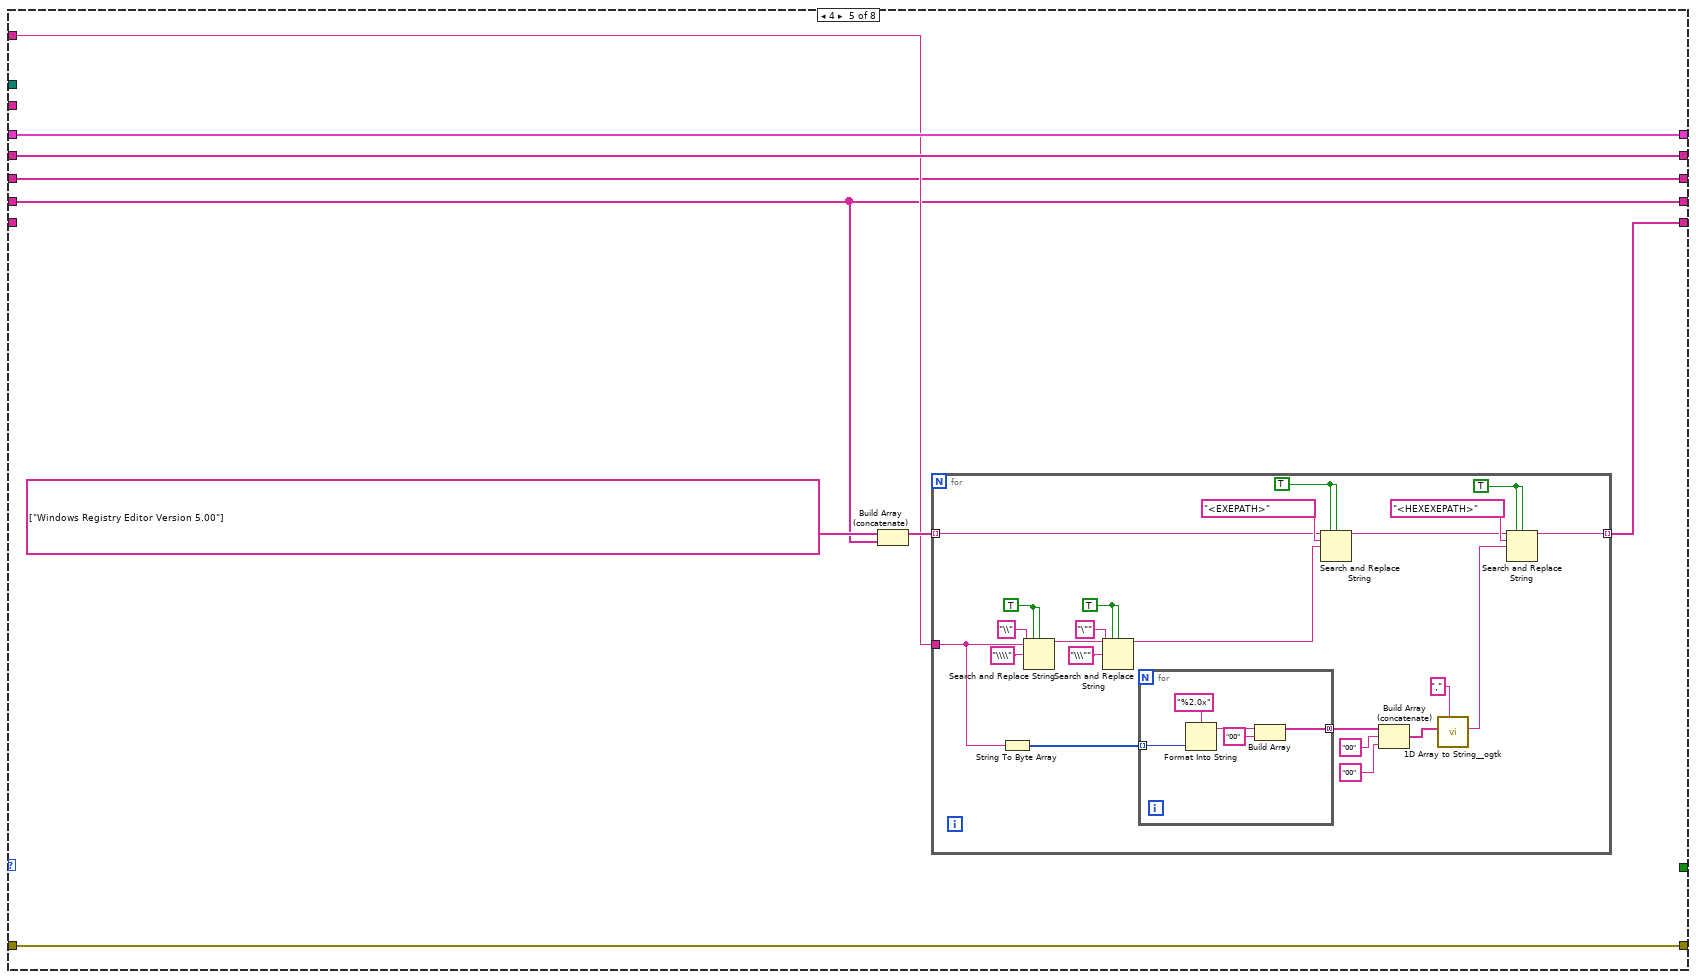
[diagram p6: hidden frame]
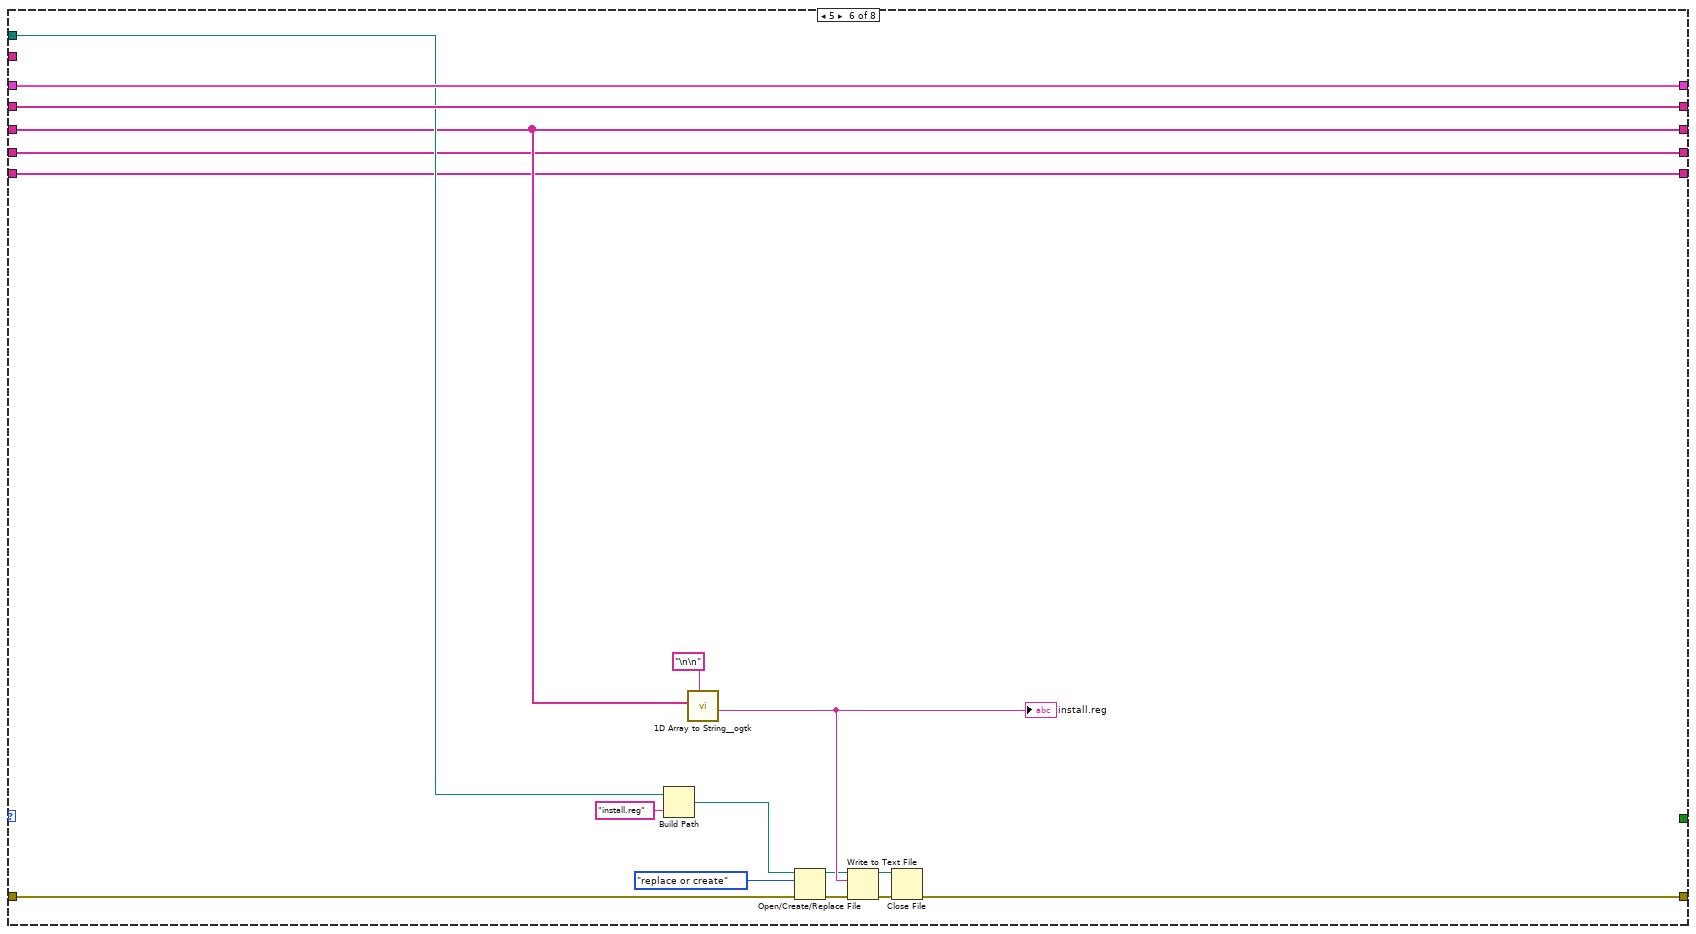
[diagram p7: hidden frame]
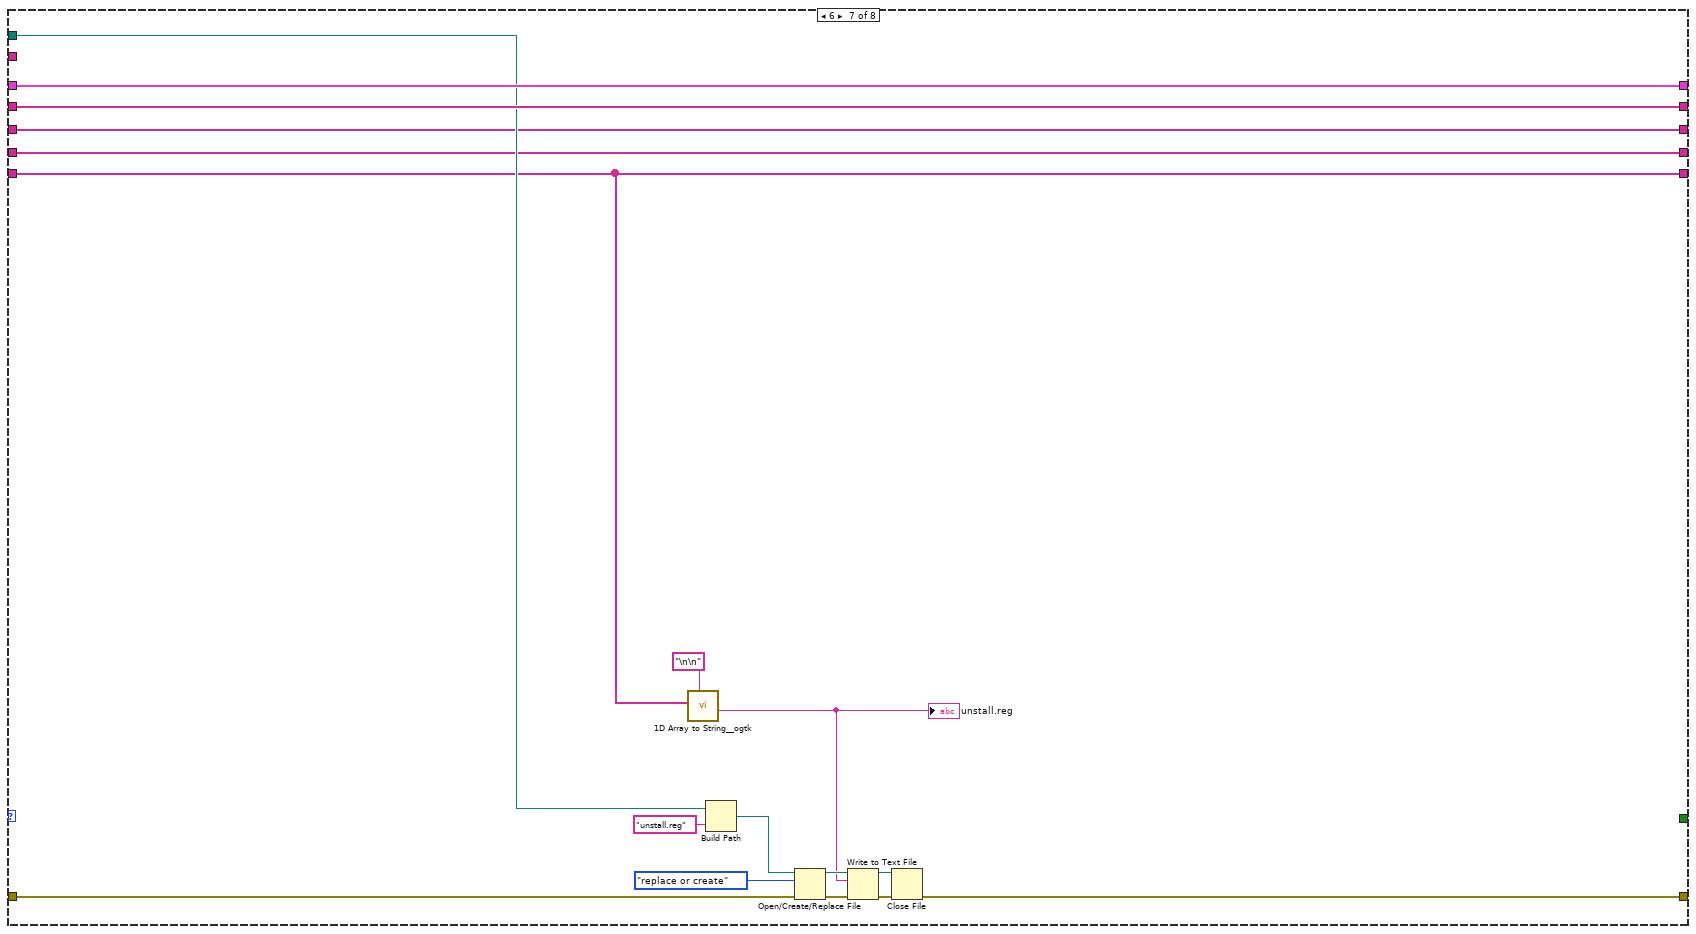
[diagram p8: hidden frame]
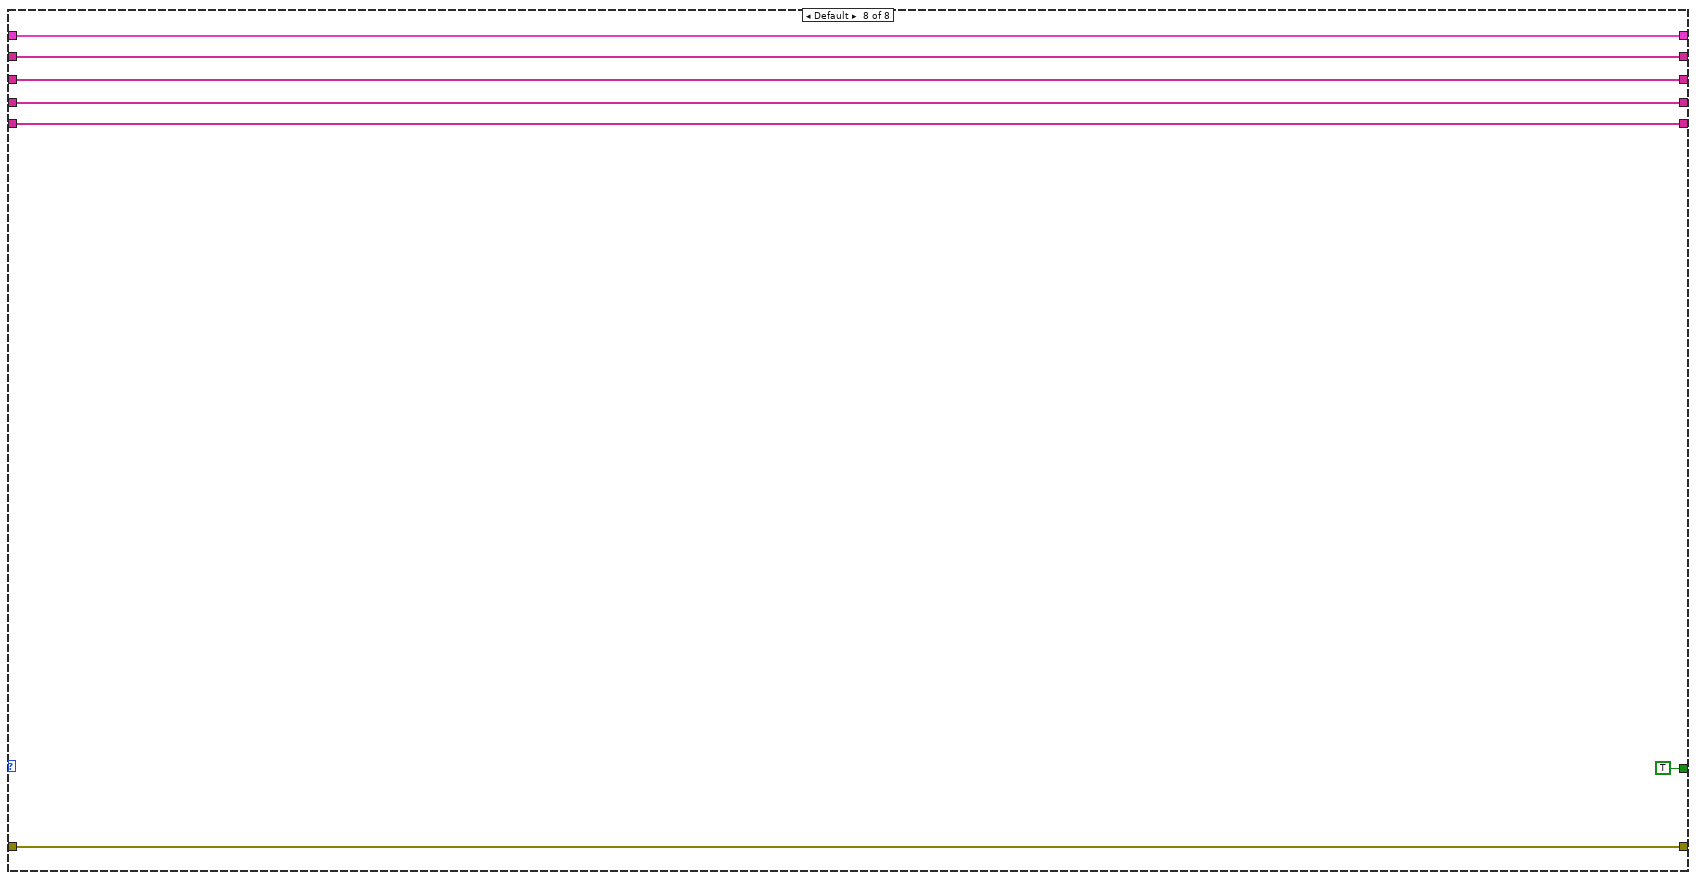
[diagram p9: hidden frame]
diagram:
  (unwired) string[] ["[HKEY_CLASSES_ROOT\\<EXTTYPE>\\shell\\open\\command]\n@=\"<EXEPATH>\"", "[HKEY_LOCAL_MACHINE\\SOFTWARE\\Classes\\<EXTTYPE>\\shell\\open\\command]\n@=hex(2):<HEXEXEPATH>", "[HKEY_CLASSES_ROOT\\<EXTTYPE>\\shell\\open\\command]\n@=\"<EXEPATH>\"", "[HKEY_CURRENT_USER\\Software\\Classes\\<EXTTYPE>\\shell\\open\\command]\n@=\"<EXEPATH>\""]
  (unwired) string[] ["[HKEY_CURRENT_USER\\Software\\Microsoft\\Windows\\CurrentVersion\\Explorer\\FileExts\\<dotEXT>\\OpenWithList]\n\"a\"=\"TDMS Viewer.exe\"\n\"MRUList\"=\"a\"", "[HKEY_CURRENT_USER\\Software\\Microsoft\\Windows\\CurrentVersion\\Explorer\\FileExts\\<dotEXT>\\OpenWithProgids]\n\"<EXTTYPE>\"=hex(2):<HEXEXEPATH>", "[-HKEY_CURRENT_USER\\Software\\Microsoft\\Windows\\CurrentVersion\\Explorer\\FileExts\\<dotEXT>\\UserChoice]", "[HKEY_CLASSES_ROOT\\<EXTTYPE>\\shell\\open\\command]\n@=\"<EXEPATH>\"", "[HKEY_LOCAL_MACHINE\\SOFTWARE\\Classes\\<EXTTYPE>\\shell\\open\\command]\n@=hex(2):<HEXEXEPATH>", "[HKEY_CLASSES_ROOT\\<EXTTYPE>\\shell\\open\\command]\n@=\"<EXEPATH>\"", "[HKEY_CURRENT_USER\\Software\\Classes\\<EXTTYPE>\\shell\\open\\command]\n@=\"<EXEPATH>\""]
  # "backup"
  n1 = Path To String(path="exe path") -> (string=w6:string)
  n2 = Format Into String(format string="\"%s\" \"%%1\"", w6) -> (resulting string=w4:string)  [unwired: 2 in, 1 out]
  n3 = while {
    tunnel: "extensions" -> [w23]
    shift-right: [w22] -> _
    shift-left: _ -> [w21]
    shift-right: [w20] -> _
    shift-left: _ -> [w19]
    tunnel: w4 -> [w18]
    shift-right: [w17] -> _
    shift-left: _ -> [w16]
    tunnel: "reg patch file" -> [w15]
    shift-right: [w13] -> w1
    shift-left: "error in" -> [w14]
    shift-right: [w12] -> _
    shift-left: _ -> [w11]
    shift-right: [w10] -> _
    shift-left: _ -> [w9]
    i -> [w25]
    stop <- w24 stop-if-true
    n4 = case shown="1" w25 {
      tunnel: [_ _ _ _ _ _ _ TRUE] -> w24
      tunnel: w23 -> [w32 _ _ _ _ _ _ _]
      tunnel: [w31 w53 w88 w123 w152 w197 w214 w221] -> w22
      tunnel: w21 -> [_ w53 w88 w123 w152 w197 w214 w221]
      tunnel: [w30 w54 w85 w119 w149 w196 w213 w220] -> w20
      tunnel: w19 -> [w30 _ w85 w119 w149 w196 w213 w220]
      tunnel: w18 -> [_ _ w84 _ w148 _ _ _]
      tunnel: [w29 w52 w83 w122 w145 w185 w203 w219] -> w17
      tunnel: w16 -> [w29 w52 _ w122 w145 w185 w203 w219]
      tunnel: w15 -> [_ _ _ _ _ w187 w205 _]
      tunnel: w14 -> [w28 w51 w82 w121 w147 w184 w202 w218]
      tunnel: [w28 w51 w82 w121 w147 w183 w201 w218] -> w13
      tunnel: [w27 w50 w81 w118 w146 w182 w199 w217] -> w12
      tunnel: w11 -> [w27 w50 w81 _ w146 w182 w199 w217]
      tunnel: [w26 w49 w80 w117 w144 w181 w198 w215] -> w10
      tunnel: w9 -> [w26 w49 w80 w117 _ w181 w198 w215]
      frame 0 {
        n5 = for {
          tunnel: w32 -> [w36] mode=indexing
          tunnel: [w34] -> w31 mode=indexing
          n6 = call "assoc.vi"("input 1"=w36) -> ("standard output"=w33:string)  [unwired: 10 in]
          n7 = Build Array(w33) -> (w38:string[])
          n8 = Match Pattern(string=w33, regular expression="^LabVIEWLabVIEW[\\s]") -> (after substring=w39:string, offset past match=w41:i32)  [unwired: 1 in, 2 out]
          n9 = Greater Or Equal To 0?(x=w41) -> (x >= 0?=w40:bool)
          n10 = case shown="True" w40 {
            tunnel: w39 -> [_ w48]
            tunnel: w38 -> [w43 w46]
            tunnel: [w43 w45] -> w37
            frame False {
            }
            frame True {
              n11 = Concatenate Strings("LabVIEW" ("string"), w48) -> (w44:string)
              n12 = Build Array (concatenate)(w46, w44) -> (w45:string[])
            }
          }
          n13 = Bundle(cluster=T1 {"dotEXT"="", "EXTTYPE"=[], "accoc"=""}, "dotEXT"=w36, "EXTTYPE"=w37, "accoc"=w33) -> (w34:T1)
        }
      }
      frame 1 {
        n14 = for {
          tunnel: string[] ["[HKEY_CURRENT_USER\\Software\\Microsoft\\Windows\\CurrentVersion\\Explorer\\FileExts\\<dotEXT>\\OpenWithList]\n\"a\"=\"TDMS Viewer.exe\"\n\"MRUList\"=\"a\"", "[-HKEY_CURRENT_USER\\Software\\Microsoft\\Windows\\CurrentVersion\\Explorer\\FileExts\\<dotEXT>\\UserChoice]", "[HKEY_CLASSES_ROOT\\<dotEXT>]\n@=\"NI-TDMS-File-Format\"", "[HKEY_CURRENT_USER\\Software\\Classes\\<dotEXT>]\n@=\"NI-TDMS-File-Format\""] -> [w60]
          tunnel: w53 -> [w59] mode=indexing
          tunnel: [w58] -> w54 mode=concatenating
          n15 = Unbundle By Name(w59) -> ("dotEXT"=w57:string, "EXTTYPE"=w56:string[])
          n16 = for {
            tunnel: w60 -> [w65]
            tunnel: [w61] -> w58 mode=concatenating
            tunnel: w57 -> [w63]
            tunnel: w56 -> [w62] mode=indexing
            n17 = for {
              tunnel: w65 -> [w75] mode=indexing
              tunnel: [w76] -> w64 mode=indexing if=w70
              tunnel: w63 -> [w69]
              tunnel: w62 -> [w68]
              w67 = TRUE ("ignore case? (F)")
              w66 = TRUE ("ignore case? (F)")
              n18 = Search and Replace String(replace all?=w67, case sensitive?=w67, input string=w75, search string="<dotEXT>", replace string=w69) -> (result string=w77:string)  [unwired: 3 in, 3 out]
              n19 = Empty String/Path?(string/path=w69) -> (empty?=w74:bool)
              n20 = Empty String/Path?(string/path=w68) -> (empty?=w73:bool)
              n21 = Not(x=w74) -> (.not. x?=w71:bool)
              n22 = Not(x=w73) -> (.not. x?=w72:bool)
              n23 = Search and Replace String(replace all?=w66, case sensitive?=w66, input string=w77, search string="<EXTTYPE>", replace string=w68) -> (result string=w76:string)  [unwired: 3 in, 3 out]
              n24 = And(x=w71, y=w72) -> (x .and. y?=w70:bool)
            }
            n25 = call-poly <userlib>:"Remove Duplicates from 1D Array__ogtk.vi"("Input Array"=w64) -> ("Output Array"=w61:string[])  [unwired: 1 out]
          }
        }
      }
      frame 2 {
        n26 = Build Array (concatenate)(string[] ["Windows Registry Editor Version 5.00", "[HKEY_CLASSES_ROOT\\Applications\\TDMS Viewer.exe]", "[HKEY_CLASSES_ROOT\\Applications\\TDMS Viewer.exe\\shell]", "[HKEY_CLASSES_ROOT\\Applications\\TDMS Viewer.exe\\shell\\open]", "[HKEY_CLASSES_ROOT\\Applications\\TDMS Viewer.exe\\shell\\open\\command]\n@=\"<EXEPATH>\"", "[HKEY_CURRENT_USER\\Software\\Classes\\Applications\\TDMS Viewer.exe]", "[HKEY_CURRENT_USER\\Software\\Classes\\Applications\\TDMS Viewer.exe\\shell]", "[HKEY_CURRENT_USER\\Software\\Classes\\Applications\\TDMS Viewer.exe\\shell\\open]", "[HKEY_CURRENT_USER\\Software\\Classes\\Applications\\TDMS Viewer.exe\\shell\\open\\command]\n@=\"<EXEPATH>\"", "[HKEY_CLASSES_ROOT\\NI-TDMS-File-Format]", "[HKEY_CLASSES_ROOT\\NI-TDMS-File-Format\\shell]", "[HKEY_CLASSES_ROOT\\NI-TDMS-File-Format\\shell\\open]", "[HKEY_CLASSES_ROOT\\NI-TDMS-File-Format\\shell\\open\\command]\n@=\"<EXEPATH>\"", "[HKEY_CURRENT_USER\\Software\\Classes\\NI-TDMS-File-Format]", "[HKEY_CURRENT_USER\\Software\\Classes\\NI-TDMS-File-Format\\shell]", "[HKEY_CURRENT_USER\\Software\\Classes\\NI-TDMS-File-Format\\shell\\open]", "[HKEY_CURRENT_USER\\Software\\Classes\\NI-TDMS-File-Format\\shell\\open\\command]\n@=\"<EXEPATH>\""], w85) -> (w86:string[])
        n27 = for {
          tunnel: w86 -> [w110] mode=indexing
          tunnel: w84 -> [w103]
          tunnel: [w105] -> w83 mode=indexing
          w89 = TRUE ("ignore case? (F)")
          w90 = TRUE ("ignore case? (F)")
          w92 = TRUE ("replace all? (F)")
          w91 = TRUE ("replace all? (F)")
          n28 = String To Byte Array(string=w103) -> (unsigned byte array=w102:u8[])
          n29 = Search and Replace String(replace all?=w91, case sensitive?=w91, input string=w103, search string="\\", replace string="\\\\" ("replace string (\"\")")) -> (result string=w94:string)  [unwired: 3 in, 3 out]
          n30 = Search and Replace String(replace all?=w92, case sensitive?=w92, input string=w94, search string="\"", replace string="\\\"" ("replace string (\"\")")) -> (result string=w93:string)  [unwired: 3 in, 3 out]
          n31 = for {
            tunnel: [w113] -> w104 mode=concatenating
            tunnel: w102 -> [w116] mode=indexing
            n32 = Format Into String(format string="%2.0x", w116) -> (resulting string=w114:string)  [unwired: 2 in, 1 out]
            n33 = Build Array(w114, "00" ("element")) -> (w113:string[])
          }
          n34 = Search and Replace String(replace all?=w90, case sensitive?=w90, input string=w110, search string="<EXEPATH>", replace string=w93) -> (result string=w106:string)  [unwired: 3 in, 3 out]
          n35 = Build Array (concatenate)(w104, "00" ("element"), "00" ("element")) -> (w99:string[])
          n36 = call <userlib>:"1D Array to String__ogtk.vi"("delimiter (Tab)"=",", "Array of Strings"=w99) -> ("delimited string"=w101:string)  [unwired: 9 in]
          n37 = Search and Replace String(replace all?=w89, case sensitive?=w89, input string=w106, search string="<HEXEXEPATH>", replace string=w101) -> (result string=w105:string)  [unwired: 3 in, 3 out]
        }
      }
      frame 3 {
        n38 = for {
          tunnel: string[] ["[-HKEY_CURRENT_USER\\Software\\Microsoft\\Windows\\CurrentVersion\\Explorer\\FileExts\\<dotEXT>\\UserChoice]", "[HKEY_CLASSES_ROOT\\<dotEXT>]\n@=\"<accoc>\"", "[HKEY_CURRENT_USER\\Software\\Classes\\<dotEXT>]\n@=\"<accoc>\""] -> [w129]
          tunnel: w123 -> [w128] mode=indexing
          tunnel: [w127] -> w118 mode=concatenating
          n39 = Unbundle By Name(w128) -> ("dotEXT"=w126:string, "accoc"=w125:string)  [unwired: 1 out]
          n40 = for {
            tunnel: w129 -> [w139] mode=indexing
            tunnel: [w140] -> w124 mode=indexing if=w134
            tunnel: w126 -> [w133]
            tunnel: w125 -> [w132]
            w131 = TRUE ("ignore case? (F)")
            w130 = TRUE ("ignore case? (F)")
            n41 = Search and Replace String(replace all?=w131, case sensitive?=w131, input string=w139, search string="<dotEXT>", replace string=w133) -> (result string=w141:string)  [unwired: 3 in, 3 out]
            n42 = Empty String/Path?(string/path=w133) -> (empty?=w138:bool)
            n43 = Empty String/Path?(string/path=w132) -> (empty?=w137:bool)
            n44 = Not(x=w138) -> (.not. x?=w135:bool)
            n45 = Not(x=w137) -> (.not. x?=w136:bool)
            n46 = Search and Replace String(replace all?=w130, case sensitive?=w130, input string=w141, search string="<accoc>", replace string=w132) -> (result string=w140:string)  [unwired: 3 in, 3 out]
            n47 = And(x=w135, y=w136) -> (x .and. y?=w134:bool)
          }
          n48 = call-poly <userlib>:"Remove Duplicates from 1D Array__ogtk.vi"("Input Array"=w124) -> ("Output Array"=w127:string[])  [unwired: 1 out]
        }
      }
      frame 4 {
        n49 = Build Array (concatenate)(string[] ["Windows Registry Editor Version 5.00"], w146) -> (w150:string[])
        n50 = for {
          tunnel: w150 -> [w174] mode=indexing
          tunnel: w148 -> [w167]
          tunnel: [w169] -> w144 mode=indexing
          w153 = TRUE ("ignore case? (F)")
          w154 = TRUE ("ignore case? (F)")
          w156 = TRUE ("replace all? (F)")
          w155 = TRUE ("replace all? (F)")
          n51 = String To Byte Array(string=w167) -> (unsigned byte array=w166:u8[])
          n52 = Search and Replace String(replace all?=w155, case sensitive?=w155, input string=w167, search string="\\", replace string="\\\\" ("replace string (\"\")")) -> (result string=w158:string)  [unwired: 3 in, 3 out]
          n53 = Search and Replace String(replace all?=w156, case sensitive?=w156, input string=w158, search string="\"", replace string="\\\"" ("replace string (\"\")")) -> (result string=w157:string)  [unwired: 3 in, 3 out]
          n54 = for {
            tunnel: [w177] -> w168 mode=concatenating
            tunnel: w166 -> [w180] mode=indexing
            n55 = Format Into String(format string="%2.0x", w180) -> (resulting string=w178:string)  [unwired: 2 in, 1 out]
            n56 = Build Array(w178, "00" ("element")) -> (w177:string[])
          }
          n57 = Search and Replace String(replace all?=w154, case sensitive?=w154, input string=w174, search string="<EXEPATH>", replace string=w157) -> (result string=w170:string)  [unwired: 3 in, 3 out]
          n58 = Build Array (concatenate)(w168, "00" ("element"), "00" ("element")) -> (w163:string[])
          n59 = call <userlib>:"1D Array to String__ogtk.vi"("delimiter (Tab)"=",", "Array of Strings"=w163) -> ("delimited string"=w165:string)  [unwired: 9 in]
          n60 = Search and Replace String(replace all?=w153, case sensitive?=w153, input string=w170, search string="<HEXEXEPATH>", replace string=w165) -> (result string=w169:string)  [unwired: 3 in, 3 out]
        }
      }
      frame 5 {
        n61 = Build Path(base path=w187, name or relative path="install.reg") -> (appended path=w186:path)
        n62 = call <userlib>:"1D Array to String__ogtk.vi"("delimiter (Tab)"="\n\n", "Array of Strings"=w185) -> ("delimited string"=w195:string)  [unwired: 9 in]
        "install.reg" <- w195
        n63 = Open/Create/Replace File(file path (use dialog)=w186, error in=w184, operation (0:open)=T2."replace or create") -> (refnum out=w191:refnum<file>, error out=w194:errorcluster)  [unwired: 3 in, 1 out]
        n64 = Write to Text File(file (use dialog)=w191, text=w195, error in=w194) -> (refnum out=w192:refnum<file>, error out=w193:errorcluster)  [unwired: 1 in, 1 out]
        n65 = Close File(refnum=w192, error in=w193) -> (error out=w183:errorcluster)  [unwired: 1 out]
      }
      frame 6 {
        n66 = call <userlib>:"1D Array to String__ogtk.vi"("delimiter (Tab)"="\n\n", "Array of Strings"=w198) -> ("delimited string"=w200:string)  [unwired: 9 in]
        "unstall.reg" <- w200
        n67 = Build Path(base path=w205, name or relative path="unstall.reg") -> (appended path=w204:path)
        n68 = Open/Create/Replace File(file path (use dialog)=w204, error in=w202, operation (0:open)=T2."replace or create") -> (refnum out=w209:refnum<file>, error out=w212:errorcluster)  [unwired: 3 in, 1 out]
        n69 = Write to Text File(file (use dialog)=w209, text=w200, error in=w212) -> (refnum out=w210:refnum<file>, error out=w211:errorcluster)  [unwired: 1 in, 1 out]
        n70 = Close File(refnum=w210, error in=w211) -> (error out=w201:errorcluster)  [unwired: 1 out]
      }
      frame Default {
      }
    }
  }
  "error out" <- w1
